vi "PhotonPoseEstimator_New_Minimal.vi"(6 "BaseNTName":string="/photonvision", 8 "RobotToCamera":T1={"TRANSLATION3D"={"X"=0.0, "Y"=0.0, "Z"=0.0}, "ROTATION3D"={"Q_quaternion"={"R"=1.0, "V"=[0.0, 0.0, 0.0]}}, "XF"=FALSE} {"TRANSLATION3D"."Z" format="%14.3f"; "TRANSLATION3D"."Y" format="%14.3f"; "TRANSLATION3D"."X" format="%14.3f"}, 9 "Camera":string, 11 "AprilTagFieldLayout":T5={"AprilTagMap"={}, "FieldLength"=0.0, "FieldWidth"=0.0, "OriginPosition "=enum."kBlueAllianceWallRightSide,", "OriginPose3d"={"Translation3d"={"X"=0.0, "Y"=0.0, "Z"=0.0}, "Rotation3d"={"Q_quaternion"={"R"=1.0, "V"=[0.0, 0.0, 0.0]}}}} {"OriginPose3d"."Translation3d"."Z" format="%14.3f"; "OriginPose3d"."Translation3d"."Y" format="%14.3f"; "OriginPose3d"."Translation3d"."X" format="%14.3f"}) -> (3 "PhotonPoseEstimator":T9={"LastPose"={"Translation3d"={"X"=0.0, "Y"=0.0, "Z"=0.0}, "Rotation3d"={"Q_quaternion"={"R"=1.0, "V"=[0.0, 0.0, 0.0]}}}, "ReferencePose"={"Translation3d"={"X"=0.0, "Y"=0.0, "Z"=0.0}, "Rotation3d"={"Q_quaternion"={"R"=1.0, "V"=[0.0, 0.0, 0.0]}}}, "FieldTags"={"AprilTagMap"={}, "FieldLength"=0.0, "FieldWidth"=0.0, "OriginPosition "=enum."kBlueAllianceWallRightSide,", "OriginPose3d"={"Translation3d"={"X"=0.0, "Y"=0.0, "Z"=0.0}, "Rotation3d"={"Q_quaternion"={"R"=1.0, "V"=[0.0, 0.0, 0.0]}}}}, "PrimaryStratety"=enum."LOWEST_AMBIGUITY", "Camera"="", "RobotToCamera"={"TRANSLATION3D"={"X"=0.0, "Y"=0.0, "Z"=0.0}, "ROTATION3D"={"Q_quaternion"={"R"=1.0, "V"=[0.0, 0.0, 0.0]}}, "XF"=FALSE}, "ReportedErrors"=[], "HighestAmbiguity"=10.0, "MultiTagFallbackStrategy"=enum."LOWEST_AMBIGUITY", "PoseCacheTimeoutSec"=-1.0, "PhotonTargetModel"={"Vertices"=[], "IsPlaner"=FALSE, "IsSpherical"=FALSE}, "BaseNTName"="/photonvision"} {"PhotonTargetModel"."Vertices"."Z" format="%14.3f"; "PhotonTargetModel"."Vertices"."Y" format="%14.3f"; "PhotonTargetModel"."Vertices"."X" format="%14.3f"; "RobotToCamera"."TRANSLATION3D"."Z" format="%14.3f"; "RobotToCamera"."TRANSLATION3D"."Y" format="%14.3f"; "RobotToCamera"."TRANSLATION3D"."X" format="%14.3f"; "FieldTags"."OriginPose3d"."Translation3d"."Z" format="%14.3f"; "FieldTags"."OriginPose3d"."Translation3d"."Y" format="%14.3f"; "FieldTags"."OriginPose3d"."Translation3d"."X" format="%14.3f"; "ReferencePose"."Translation3d"."Z" format="%14.3f"; "ReferencePose"."Translation3d"."Y" format="%14.3f"; "ReferencePose"."Translation3d"."X" format="%14.3f"; "LastPose"."Translation3d"."Z" format="%14.3f"; "LastPose"."Translation3d"."Y" format="%14.3f"; "LastPose"."Translation3d"."X" format="%14.3f"})   [LabVIEW 2019, in "PhotonVisionLib.lvlib"]
doc: "Create a new Photon Pose Estimator data cluster.\n\nThe PhotonPoseEstimator functions filters or combines readings from all the AprilTags visible at a given timestamp on the field to produce a single robot in field pose, using the strategy set below. Example usage can be found under the LabVIEW Find Examples..\n\nInputs:\n -- AprilTagFieldLayout -- cluster -- A WPILib LabVIEW Math cluster defining the absolute positions of April Tags on a FIRST field. with respect to the FIRST field \n -- Strategy -- Enum -- The strategy it should use to determine the best pose. Current strategies include:\n LOWEST_AMBIGUITY -- Choose the Pose with the lowest ambiguity\n CLOSEST_TO_CAMERA_HEIGHT -- Choose the Pose which is closest to the camera height.\n CLOSEST_TO_REFERENCE_POSE -- Choose the Pose which is closest to a set Reference position.\n CLOSEST_TO_LAST_POSE -- Choose the Pose which is closest to the last pose calculated\n AVERAGE_BEST_TARGETS -- Weight average of acceptable targets based on ambiguity..\n -- CameraName -- String -- Name of the photon camera.\n -- RobotToCamera -- Transform3d -- Transform from the center of the robot to the camera mount positions\n\nOutputs:\n -- PhotonPoseEstimator -- cluster -- created data cluster."
uses:
  TypeDef/PhotonPoseEstimatorType.ctl
  <vilib>/Rock Robotics/WPI/ThirdParty/JAS_Junk/TrajLib/TypeDef/POSE3D.ctl
  <vilib>/Rock Robotics/WPI/ThirdParty/JAS_Junk/TrajLib/TypeDef/TRANSLATION3D.ctl
  <vilib>/Rock Robotics/WPI/ThirdParty/JAS_Junk/TrajLib/TypeDef/ROTATION3D.ctl
  <vilib>/Rock Robotics/WPI/ThirdParty/JAS_Junk/TrajLib/TypeDef/QUATERNION.ctl
  <vilib>/Rock Robotics/WPI/ThirdParty/JAS_Junk/TrajLib/TypeDef/AprilTagFieldLayout.ctl
  <vilib>/Rock Robotics/WPI/ThirdParty/JAS_Junk/TrajLib/TypeDef/AprilTag.ctl
  <vilib>/Rock Robotics/WPI/ThirdParty/JAS_Junk/TrajLib/Enum/AprilTagFieldLayoutOrignPosition_ENUM.ctl
  Enum/PhotonPoseStrategy_ENUM.ctl
  <vilib>/Rock Robotics/WPI/ThirdParty/JAS_Junk/TrajLib/TypeDef/TRANSFORM3D.ctl
  TypeDef/PhotonTargetModel.ctl
  PhotonTargetModel_New_RectPlanar.vi
  <vilib>/Rock Robotics/WPI/ThirdParty/JAS_Junk/TrajLib/Conv_Inches_Meters.vi
  <vilib>/Rock Robotics/WPI/ThirdParty/JAS_Junk/TrajLib/VI/Translation3d_Create.vi
  PhotonTargetModel_New.vi
  PhotonVision_Globals.vi
  PhotonVisionLib.lvlib
  <vilib>/Rock Robotics/WPI/ThirdParty/JAS_Junk/TrajLib/Trajectory_Library.lvlib
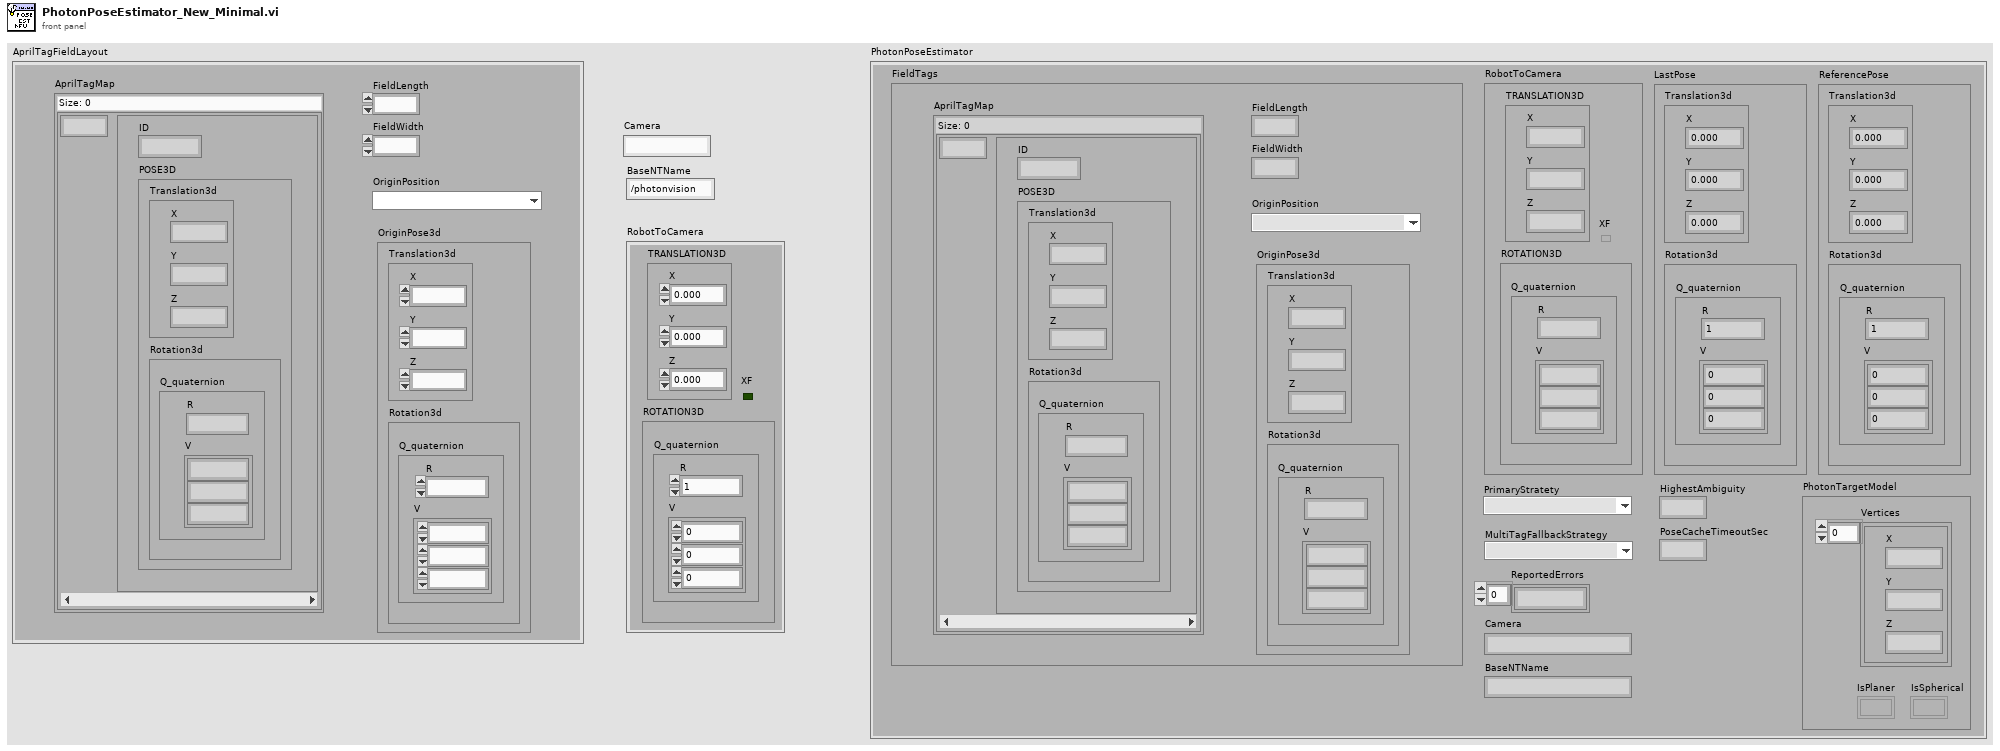
[diagram p1: front panel]
types:
  T1 = typedef "Trajectory_Library.lvlib/TRANSFORM3D.ctl" = cluster{"TRANSLATION3D":T2, "ROTATION3D":T3, "XF":bool}
  T2 = typedef "Trajectory_Library.lvlib/TRANSLATION3D.ctl" = cluster{"X":dbl, "Y":dbl, "Z":dbl}
  T3 = typedef "Trajectory_Library.lvlib/ROTATION3D.ctl" = cluster{"Q_quaternion":T4}
  T4 = typedef "Trajectory_Library.lvlib/QUATERNION.ctl" = cluster{"R":dbl, "V":dbl[]}
  T5 = typedef "Trajectory_Library.lvlib/AprilTagFieldLayout.ctl" = cluster{"AprilTagMap":map{i32, T6}, "FieldLength":dbl, "FieldWidth":dbl, "OriginPosition ":T8, "OriginPose3d":T7}
  T6 = typedef "Trajectory_Library.lvlib/AprilTag.ctl" = cluster{"ID":i32, "POSE3D":T7}
  T7 = typedef "Trajectory_Library.lvlib/POSE3D.ctl" = cluster{"Translation3d":T2, "Rotation3d":T3}
  T8 = typedef "Trajectory_Library.lvlib/AprilTagFieldLayoutOrignPosition_ENUM.ctl" = enum16{"kBlueAllianceWallRightSide,", "kRedAllianceWallRightSide,"}
  T9 = typedef "PhotonVisionLib.lvlib/PhotonPoseEstimatorType.ctl" = cluster{"LastPose":T7, "ReferencePose":T7, "FieldTags":T5, "PrimaryStratety":T10, "Camera":string, "RobotToCamera":T1, "ReportedErrors":dbl[], "HighestAmbiguity":dbl, "MultiTagFallbackStrategy":T10, "PoseCacheTimeoutSec":dbl, "PhotonTargetModel":T11, "BaseNTName":string}
  T10 = typedef "PhotonVisionLib.lvlib/PhotonPoseStrategy_ENUM.ctl" = enum16{"LOWEST_AMBIGUITY", "CLOSEST_TO_CAMERA_HEIGHT", "CLOSEST_TO_REFERENCE_POSE", "CLOSEST_TO_LAST_POSE", "AVERAGE_BEST_TARGETS", "MULTI_TAG_PNP_ON_COPROCESSOR", "MULTI_TAG_PNP_ON_RIO", "PNP_DISTANCE_TRIG_SOLVE", "CONSTRAINED_SOLVEPNP"}
  T11 = typedef "PhotonVisionLib.lvlib/PhotonTargetModel.ctl" = cluster{"Vertices":T2[], "IsPlaner":bool, "IsSpherical":bool}
  T12 = typedef "Trajectory_Library.lvlib/TIME_INTERPOLATABLE_ROTATION2D.ctl" = cluster{"TimeStamps":dbl[], "RotationValues":T13[], "Min_TimeStamp":dbl, "Max_TimeStamp":dbl, "ItemCount":i32, "MaxBufferTime":dbl}
  T13 = typedef "Trajectory_Library.lvlib/ROTATION2D.ctl" = cluster{"VALUE":dbl, "COS":dbl, "SIN":dbl}
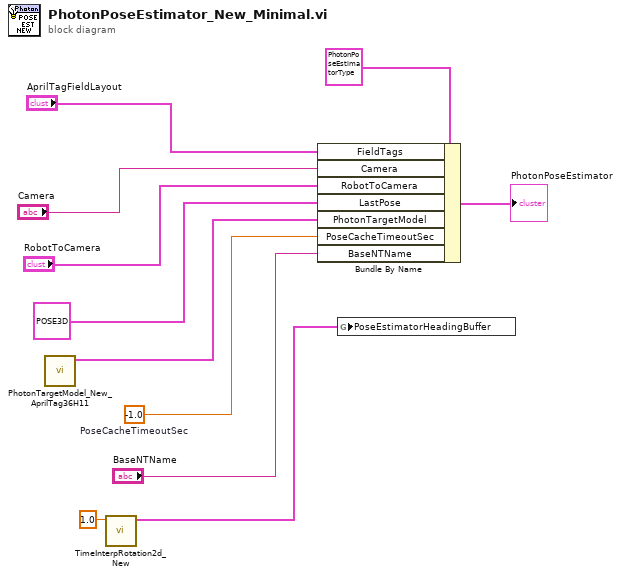
[diagram p0: block diagram]
diagram:
  w5 = -1.0  # PoseCacheTimeoutSec
  n1 = call "PhotonTargetModel_New_AprilTag36H11.vi"() -> ("PhotonTargetModel"=w3:T11)  [unwired: 11 in]
  n2 = call <vilib>:"TimeInterpRotation2d_New.vi"("MaxTime"=1.0) -> ("TimeInterpRotation"=w1:T12)  [unwired: 10 in]
  n3 = Bundle By Name(cluster=T9 {"LastPose"={"Translation3d"={"X"=0.0, "Y"=0.0, "Z"=0.0}, "Rotation3d"={"Q_quaternion"={"R"=1.0, "V"=[0.0, 0.0, 0.0]}}}, "ReferencePose"={"Translation3d"={"X"=0.0, "Y"=0.0, "Z"=0.0}, "Rotation3d"={"Q_quaternion"={"R"=1.0, "V"=[0.0, 0.0, 0.0]}}}, "FieldTags"={"AprilTagMap"={}, "FieldLength"=0.0, "FieldWidth"=0.0, "OriginPosition "=enum."kBlueAllianceWallRightSide,", "OriginPose3d"={"Translation3d"={"X"=0.0, "Y"=0.0, "Z"=0.0}, "Rotation3d"={"Q_quaternion"={"R"=1.0, "V"=[0.0, 0.0, 0.0]}}}}, "PrimaryStratety"=enum."LOWEST_AMBIGUITY", "Camera"="", "RobotToCamera"={"TRANSLATION3D"={"X"=0.0, "Y"=0.0, "Z"=0.0}, "ROTATION3D"={"Q_quaternion"={"R"=1.0, "V"=[0.0, 0.0, 0.0]}}, "XF"=FALSE}, "ReportedErrors"=[], "HighestAmbiguity"=0.3, "MultiTagFallbackStrategy"=enum."LOWEST_AMBIGUITY", "PoseCacheTimeoutSec"=-1.0, "PhotonTargetModel"={"Vertices"=[], "IsPlaner"=FALSE, "IsSpherical"=FALSE}, "BaseNTName"="/photonvision"} ("PhotoPoseEstimator"), "FieldTags"="AprilTagFieldLayout", "Camera"="Camera", "RobotToCamera"="RobotToCamera", "LastPose"=T7 {"Translation3d"={"X"=0.0, "Y"=0.0, "Z"=0.0}, "Rotation3d"={"Q_quaternion"={"R"=1.0, "V"=[0.0, 0.0, 0.0]}}}, "PhotonTargetModel"=w3, "PoseCacheTimeoutSec"=w5, "BaseNTName"="BaseNTName") -> (→"PhotonPoseEstimator":T9)
  n4 = global write "PhotonVision_Globals.vi" "PoseEstimatorHeadingBuffer"(w1) -> ()
